vi "Exercise 1.vi"   [LabVIEW 2014, in "Singh_Patel_3rd_Exercise1_12-2-16.lvrbt"]
uses:
  Singh_Patel_3rd_Exercise1_12-2-16.lvrbt
  <vilib>/NXT/Block Support/NXT_OutputPort.ctl
  <vilib>/NXT/NXTIO Xnodes/NXTIONodeSubVIs/NXTMoveMotors.vi
  <vilib>/NXT/Subs/LVHSConnector.ctl
  <vilib>/NXT/NXTIO Xnodes/AddressXNode/NXTIOAddress.xnode
  <vilib>/NXT/NXTIO Xnodes/NXTIOXNode/NXTIO.xnode
  <vilib>/NXT/LegoClasses/BrickReference/BrickReference.lvclass
types:
  T1 = typedef "NXT_OutputPort.ctl" = u8
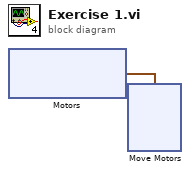
[diagram p0: block diagram]
diagram:
  n1 = xnode "Motors"() -> ("Motor"=w1:cluster{"Port":T1, "Port":T1})
  n2 = xnode "Move Motors"("Motors"=w1) -> ()  [unwired: 3 in, 1 out]
